vi "DSF.Engine.Runtime.Create.vi"(7 "id":i32, 8 "error in (no error)":errorcluster, 10 "Timing":refnum<class "DSF.Shared.Timing.lvclass">, 11 "DSF Runtime in":refnum<class "DSF.Engine.Runtime.lvclass">) -> (0 "error out":errorcluster, 3 "DSF Runtime out":refnum<class "DSF.Engine.Runtime.lvclass">)   [LabVIEW 2017, in "DSF.Engine.lvlib" / "DSF.Engine.Runtime.lvclass"]
uses:
  DSF.Engine.Runtime.lvclass
  Shared/Classes/Timing/DSF.Shared.Timing.lvclass
  DSF.Engine.Runtime.lvclass/DSF.Engine.Runtime.ctl
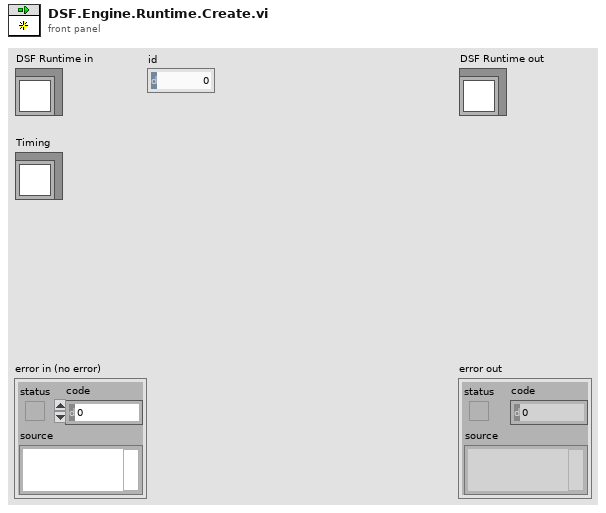
[diagram p1: front panel]
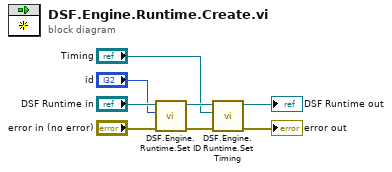
[diagram p0: block diagram]
diagram:
  n1 = call "DSF.Engine.Runtime.Set ID.vi"("error in (no error)"="error in (no error)", "id"="id", "Runtime in"="DSF Runtime in") -> ("error out"=w6:errorcluster, "Runtime out"=w5:refnum<class "DSF.Engine.Runtime.lvclass">)  [unwired: 7 in]
  n2 = call "DSF.Engine.Runtime.Set Timing.vi"("error in (no error)"=w6, "Timing"="Timing", "Runtime in"=w5) -> ("error out"=→"error out":errorcluster, "Runtime out"=→"DSF Runtime out":refnum<class "DSF.Engine.Runtime.lvclass">)  [unwired: 7 in]
